vi "Loop test.vi"() -> ()   [LabVIEW 2019]
panel:
  out "x-y":u32
  in  "Stop Button":bool
  out "Waveform Chart":dbl[][](graph)
  in  "VISA resource name":refnum<visa-resource-name>
  in  "Numeric":i32
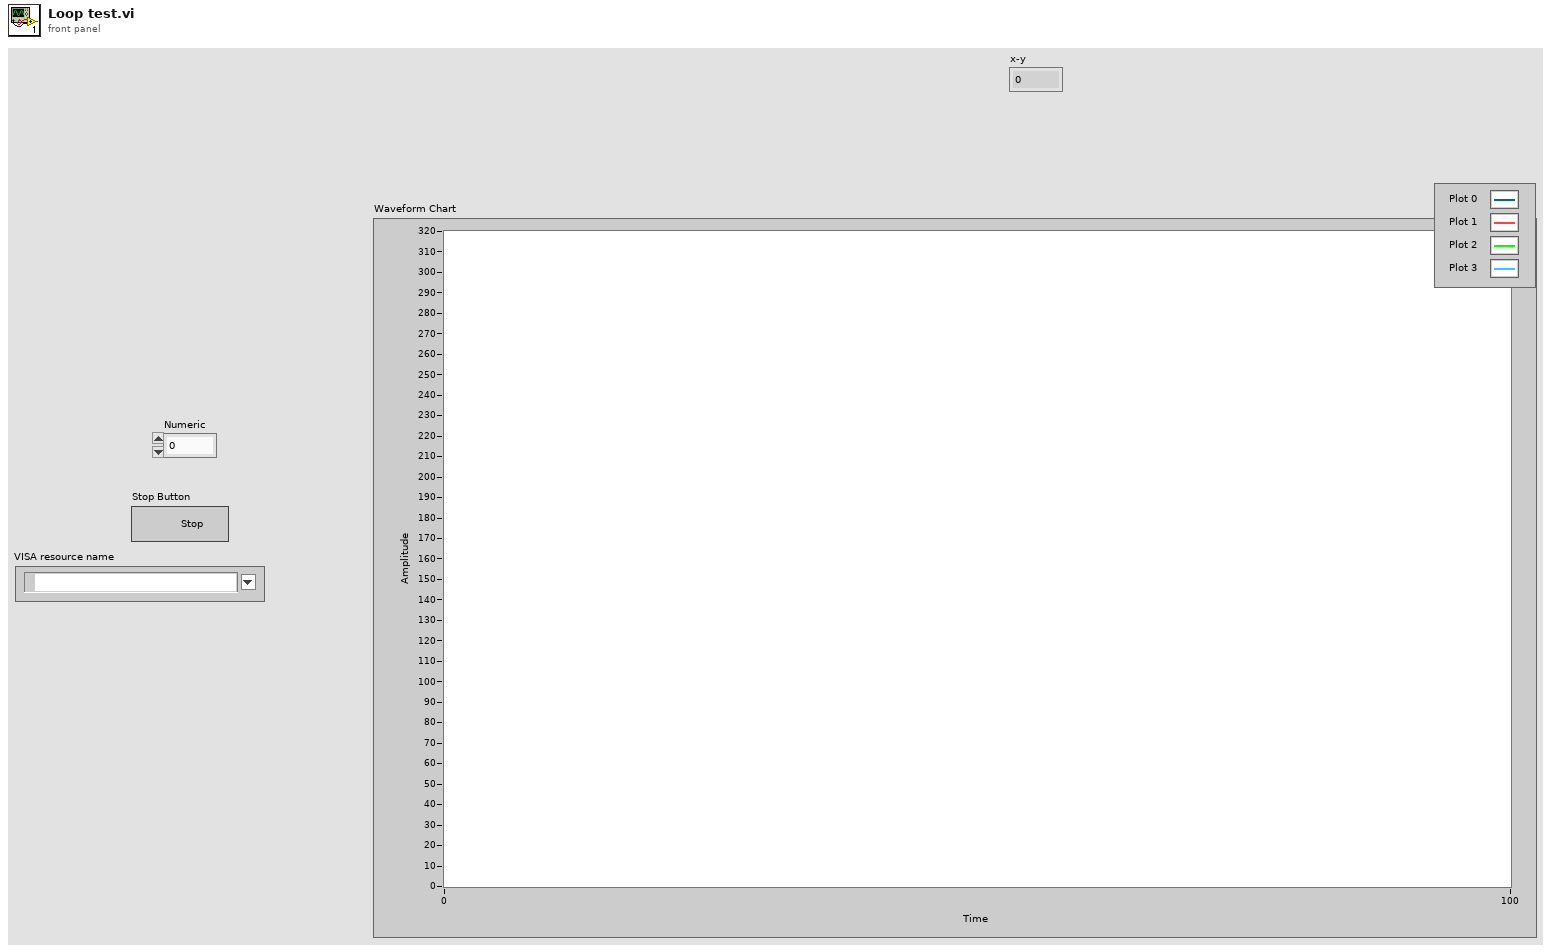
[diagram p1: front panel]
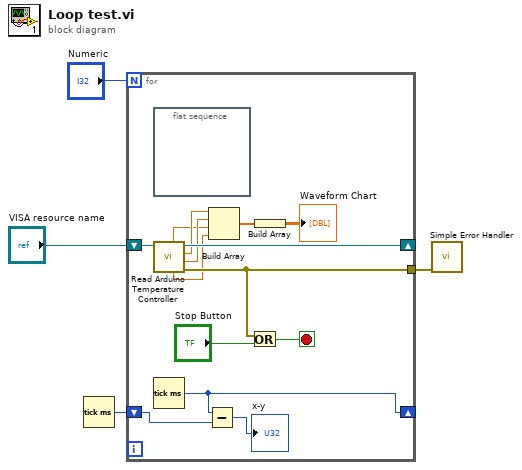
[diagram p0: block diagram]
diagram:
  n1 = Tick Count (ms)() -> (millisecond timer value=w1:u32)
  n2 = for {
    N: "Numeric" -> [_]
    tunnel: [w17] -> w2
    shift-right: [w16] -> _
    shift-left: "VISA resource name" -> [w18]
    shift-right: [w5] -> _
    shift-left: w1 -> [w6]
    stop <- w9 stop-if-true
    n3 = flat-sequence {
      frame #0 {
      }
    }
    n4 = call "Read Arduino Temperature Controller.vi"("VISA resource name"=w18) -> ("Error Out"=w17:errorcluster, "Control temperature"=w14:dbl, "Sample temperature"=w15:dbl, "VISA resource name out"=w16:refnum<visa-resource-name>, "Power"=w13:dbl, "Set point"=w12:dbl)  [unwired: 5 in]
    n5 = Tick Count (ms)() -> (millisecond timer value=w5:u32)
    n6 = Subtract(x=w5, y=w6) -> (x-y=→"x-y":u32)
    n7 = Build Array(w15, w14, w12, w13) -> (w11:dbl[])
    n8 = Or(x=w17, y="Stop Button") -> (x .or. y?=w9:bool)
    n9 = Build Array(w11) -> (→"Waveform Chart":dbl[][])
  }
  n10 = call <vilib>:"Simple Error Handler.vi"("error in (no error)"=w2) -> ()  [unwired: 4 in, 5 out]
